vi "Initialize.vi"(8 "error in (no error)":errorcluster, 11 "MFC in":refnum<class "MFC.lvclass">) -> (0 "error out":errorcluster, 3 "MFC out":refnum<class "MFC.lvclass">)   [LabVIEW 2013, in "MFC.LVLIB" / "MFC.lvclass"]
uses:
  MFC.lvclass
  <vilib>/Instr/_visa.llb/VISA Flush IO Buffer Mask.ctl
  <vilib>/Instr/_visa.llb/VISA Configure Serial Port (Instr).vi
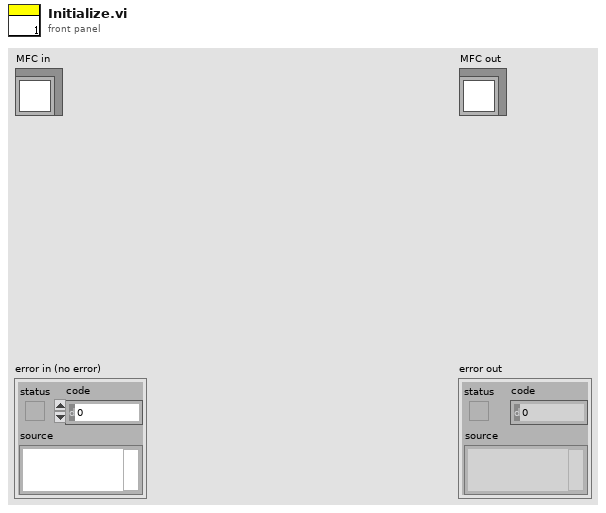
[diagram p1: front panel]
types:
  T1 = enum16{"open", "open or create", "create or replace", "create", "open (read-only)"}
  T2 = typedef "VISA Flush IO Buffer Mask.ctl" = u16
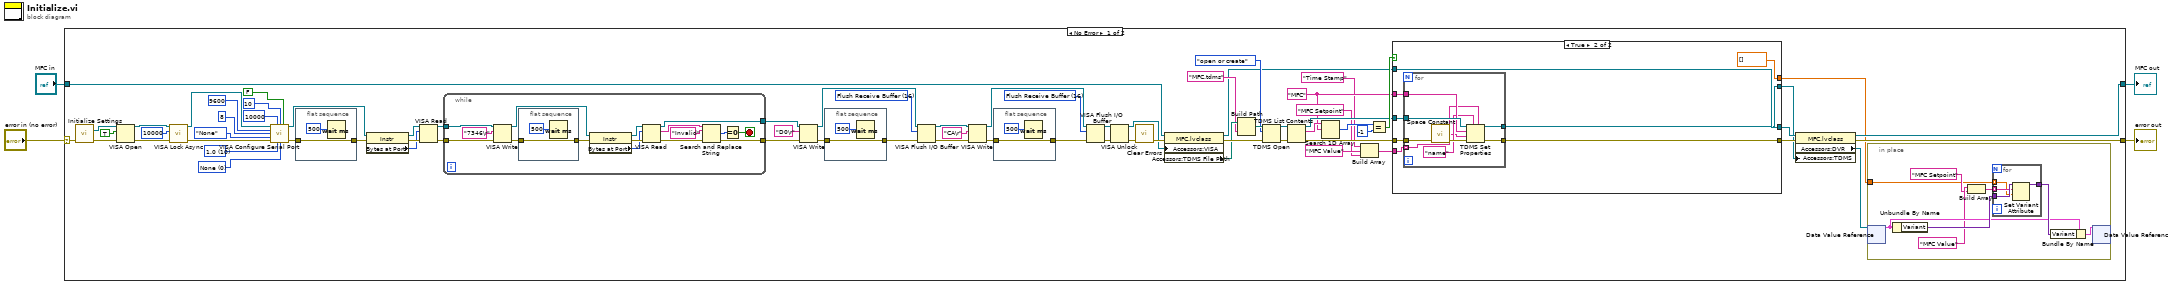
[diagram p0: block diagram]
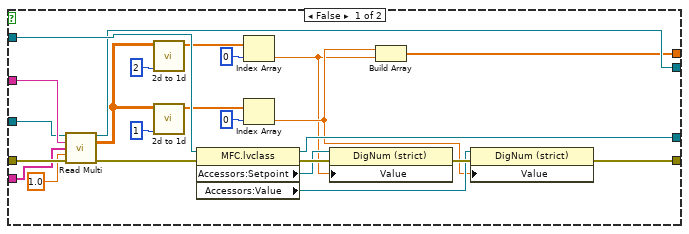
[diagram p2: hidden frame]
diagram:
  n1 = case shown="No Error" "error in (no error)" {
    selector: "error in (no error)" -> [w24 w153]
    tunnel: [w19 w153] -> w3
    tunnel: [w20 w152] -> w1
    tunnel: "MFC in" -> [w64 w152]
    frame No Error {
      w33 = T2 16 items=["Flush Receive Buffer"=16, "Write Transmit Buffer to Device"=32, "Flush Receive Buffer (No I/O)"=64, "Flush Transmit Buffer"=128] ("Mask")
      w38 = T2 16 items=["Flush Receive Buffer"=16, "Write Transmit Buffer to Device"=32, "Flush Receive Buffer (No I/O)"=64, "Flush Transmit Buffer"=128] ("Mask")
      w41 = u16 0 items=["None", "XON/XOFF", "RTS/CTS", "XON/XOFF & RTS/CTS", "DTR/DSR", "XON/XOFF & DTR/DSR"] ("flow control (0:none)")
      w42 = u16 10 items=["1.0"=10, "1.5"=15, "2.0"=20] ("stop bits (10: 1 bit)")
      w69 = "MFC"
      n2 = call "Initialize Settings.vi"("error in (no error)"=w24) -> ("VISA resource name 2"=w13:refnum<visa-resource-name>, "error out"=w14:errorcluster)  [unwired: 13 in]
      n3 = VISA Open(duplicate session (F)=TRUE, error in (no error)=w14, VISA resource name=w13) -> (VISA resource name=w16:refnum<visa-resource-name>, error out=w17:errorcluster)  [unwired: 2 in]
      n4 = call <vilib>:"VISA Lock Async.vi"("error in (no error)"=w17, "timeout (0)"=u32 10000, "VISA resource name"=w16) -> ("error out"=w11:errorcluster, "VISA resource name out"=w12:refnum<visa-resource-name>)  [unwired: 6 in, 1 out]
      n5 = call-poly "VISA Configure Serial Port"("VISA resource name"=w12, "timeout (10sec)"=u32 10000, "termination char\n(0xA = '\\n' = LF)"=u8 10 ("termination char\n(0xA = '\\n' = LF)"), "Enable Termination\nChar (T)"=FALSE ("Enable Termination\nChar (T)"), "baud rate (9600)"=u32 9600, "data bits (8)"=u16 8, "parity (0:none)"=enum16{"None", "Odd", "Even", "Mark", "Space"}."None", "error in (no error)"=w11, "stop bits (10: 1 bit)"=w42, "flow control (0:none)"=w41) -> ("VISA resource name out"=w62:refnum<visa-resource-name>, "error out"=w58:errorcluster)  [unwired: 4 in]
      n6 = flat-sequence {
        tunnel: w58 -> [w110]
        tunnel: [w110] -> w57
        frame #0 {
          n7 = Wait (ms)(milliseconds to wait=u32 500) -> ()  [unwired: 1 out]
        }
      }
      n8 = property class="Instr"(reference=w62, error in=w57) -> (reference out=w61:refnum<visa-resource-name>, error out=w60:errorcluster, "Bytes at Port"=w59:u32)
      n9 = VISA Read(VISA resource name=w61, byte count=w59, error in (no error)=w60) -> (VISA resource name out=w55:refnum<visa-resource-name>, error out=w56:errorcluster)  [unwired: 2 out]
      n10 = while {
        tunnel: w56 -> [w92]
        tunnel: w55 -> [w104]
        tunnel: [w107] -> w51
        tunnel: [w106] -> w52
        stop <- w105 stop-if-true
        n11 = VISA Write(VISA resource name=w104, write buffer="7346\r", error in (no error)=w92) -> (VISA resource name out=w102:refnum<visa-resource-name>, error out=w99:errorcluster)  [unwired: 1 out]
        n12 = flat-sequence {
          tunnel: [w108] -> w100
          tunnel: w99 -> [w108]
          frame #0 {
            n13 = Wait (ms)(milliseconds to wait=u32 500) -> ()  [unwired: 1 out]
          }
        }
        n14 = property class="Instr"(reference=w102, error in=w100) -> (reference out=w103:refnum<visa-resource-name>, error out=w101:errorcluster, "Bytes at Port"=w97:u32)
        n15 = VISA Read(VISA resource name=w103, byte count=w97, error in (no error)=w101) -> (VISA resource name out=w106:refnum<visa-resource-name>, read buffer=w93:string, error out=w94:errorcluster)  [unwired: 1 out]
        n16 = Search and Replace String(input string=w93, search string="Invalid", error in=w94) -> (number of replacements=w96:i32, error out=w107:errorcluster)  [unwired: 5 in, 2 out]
        n17 = Equal To 0?(x=w96) -> (x = 0?=w105:bool)
      }
      n18 = VISA Write(VISA resource name=w52, write buffer="D0\r", error in (no error)=w51) -> (VISA resource name out=w39:refnum<visa-resource-name>, error out=w49:errorcluster)  [unwired: 1 out]
      n19 = flat-sequence {
        tunnel: [w90] -> w40
        tunnel: w49 -> [w90]
        frame #0 {
          n20 = Wait (ms)(milliseconds to wait=u32 500) -> ()  [unwired: 1 out]
        }
      }
      n21 = VISA Flush I/O Buffer(VISA resource name=w39, mask (16)=w38, error in (no error)=w40) -> (VISA resource name out=w36:refnum<visa-resource-name>, error out=w37:errorcluster)
      n22 = VISA Write(VISA resource name=w36, write buffer="CA\r", error in (no error)=w37) -> (VISA resource name out=w34:refnum<visa-resource-name>, error out=w47:errorcluster)  [unwired: 1 out]
      n23 = flat-sequence {
        tunnel: [w88] -> w35
        tunnel: w47 -> [w88]
        frame #0 {
          n24 = Wait (ms)(milliseconds to wait=u32 500) -> ()  [unwired: 1 out]
        }
      }
      n25 = VISA Flush I/O Buffer(VISA resource name=w34, mask (16)=w33, error in (no error)=w35) -> (VISA resource name out=w9:refnum<visa-resource-name>, error out=w10:errorcluster)
      n26 = VISA Unlock(8:w10, 11:w9) -> (0:w8:errorcluster, 3:w7:refnum<visa-resource-name>)
      n27 = call <vilib>:"Clear Errors.vi"("error in (no error)"=w8) -> ("error out"=w63:errorcluster)  [unwired: 6 in]
      n28 = property class="MFC.lvclass"(reference=w64, error in=w63, "Accessors:VISA"=w7) -> (reference out=w25:refnum<class "MFC.lvclass">, error out=w31:errorcluster, "Accessors:TDMS File Path"=w28:path)
      n29 = Build Path(base path=w28, name or relative path="MFC.tdms") -> (appended path=w32:path)
      n30 = TDMS Open(8:w31, 10:T1."open or create" ("operation (0:open)"), 11:w32) -> (0:w30:errorcluster, 3:w26:refnum<k34>)  [unwired: 4 in]
      n31 = TDMS List Contents(4:w30, 7:w26) -> (0:w70:errorcluster, 2:w73:string[], 3:w71:refnum<k34>)  [unwired: 1 in, 1 out]
      n32 = Search 1D Array(1D array=w73, element=w69) -> (index of element=w74:i32)  [unwired: 1 in]
      n33 = Build Array("Time Stamp" ("Channel"), "MFC Value" ("string"), "MFC Setpoint" ("string")) -> (w68:string[])
      n34 = Equal?(x=w74, y=-1) -> (x = y?=w72:bool)
      n35 = case shown="True" w72 {
        tunnel: w71 -> [w128 w143]
        tunnel: [w118 w139] -> w22
        tunnel: w70 -> [w131 w141]
        tunnel: w69 -> [w132 w142]
        tunnel: w25 -> [w135 w138]
        tunnel: w68 -> [w116 w140]
        tunnel: [w127 w138] -> w21
        tunnel: [w115 w137] -> w6
        tunnel: [w112 dbl[] []] -> w5
        frame False {
          n36 = call "Read Multi.vi"("tdms file in"=w128, "group"=w132, "Channel"=w116, "Numeric"=1.0, "error in (no error)"=w131) -> ("tdms file out"=w115:refnum<k34>, "Array"=w125:dbl[][], "error out"=w130:errorcluster)  [unwired: 7 in, 1 out]
          n37 = call "2d to 1d.vi"("index"=2, "array"=w125) -> ("output array"=w133:dbl[])  [unwired: 9 in]
          n38 = call "2d to 1d.vi"("index"=1, "array"=w125) -> ("output array"=w124:dbl[])  [unwired: 9 in]
          n39 = property class="MFC.lvclass"(reference=w135, error in=w130) -> (reference out=w127:refnum<class "MFC.lvclass">, error out=w123:errorcluster, "Accessors:Setpoint"=w121:refnum<vi>, "Accessors:Value"=w117:refnum<vi>)
          n40 = Index Array(array=w133, index=0) -> (element=w113:dbl)
          n41 = Index Array(array=w124, index=0) -> (element=w114:dbl)
          n42 = property class="DigNum (strict)"(reference=w121, error in=w123, "Value"=w113) -> (error out=w122:errorcluster)  [unwired: 1 out]
          n43 = Build Array(w114, w113) -> (w112:dbl[])
          n44 = property class="DigNum (strict)"(reference=w117, error in=w122, "Value"=w114) -> (error out=w118:errorcluster)  [unwired: 1 out]
        }
        frame True {
          n45 = for {
            tunnel: w141 -> [w151]
            tunnel: [w150] -> w139
            tunnel: w143 -> [w149]
            tunnel: w142 -> [w148]
            tunnel: w140 -> [w147] mode=indexing
            tunnel: [w144] -> w137
            n46 = call <vilib>:"Space Constant.vi"() -> ("String"=w145:string)
            n47 = TDMS Set Properties(5:w147, 7:"name" ("property names"), 8:w151, 9:w145, 10:w148, 11:w149) -> (0:w150:errorcluster, 3:w144:refnum<k34>)  [unwired: 2 out]
          }
        }
      }
      n48 = property class="MFC.lvclass"(reference=w21, error in=w22, "Accessors:TDMS"=w6) -> (reference out=w20:refnum<class "MFC.lvclass">, error out=w19:errorcluster, "Accessors:DVR"=w23:refnum<data-value>)
      n49 = in-place {
        in-place-border: w5 -> [w76]
        n50 = in-place-dvr #1(w23) -> (w80:cluster{"Array":string[], "Variant":variant})  [unwired: 1 out]
        n51 = Unbundle By Name(w80) -> ("Variant"=w82:variant)
        n52 = Build Array("MFC Value" ("string"), "MFC Setpoint" ("string")) -> (w77:string[])
        n53 = for {
          tunnel: w82 -> [w87]
          tunnel: [w86] -> w81
          tunnel: w77 -> [w85] mode=indexing
          tunnel: w76 -> [w84] mode=indexing
          n54 = Set Variant Attribute(Variant=w87, name=w85, value=w84) -> (Variant out=w86:variant)  [unwired: 1 in, 2 out]
        }
        n55 = Bundle By Name(cluster=w80, "Variant"=w81) -> (w83:cluster{"Array":string[], "Variant":variant})
        n56 = in-place-dvr #1(w83) -> ()  [unwired: 2 out]
      }
    }
    frame Error {
    }
  }
  "error out" <- w3
  "MFC out" <- w1
